vi "Configure Module.vi"(8 "error in (no error)":errorcluster, 10 "IOV ref in":variant, 11 "Modules.lvlib:9242.lvclass":refnum<class "9242.lvclass">) -> (0 "error out":errorcluster, 2 "IOV ref out":variant, 3 "Modules.lvlib:9242.lvclass":refnum<class "9242.lvclass">)   [LabVIEW 2020, in "Modules.lvlib" / "9242.lvclass"]
uses:
  9242.lvclass
  <resource>/objmgr/cRIO.rc
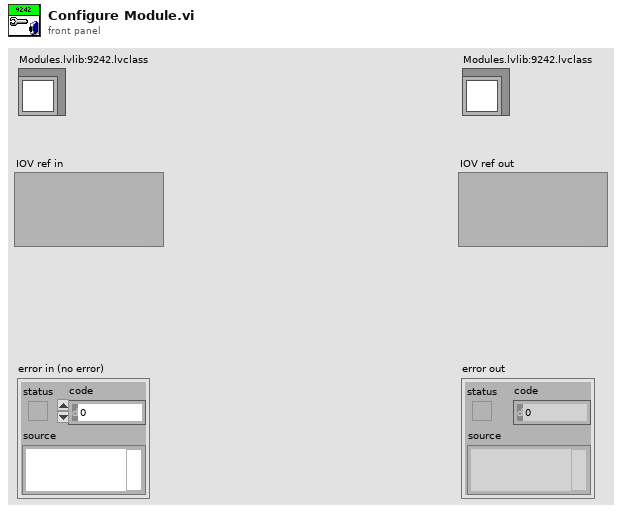
[diagram p1: front panel]
types:
  T1 = typedef "Modules.lvlib/9233.lvclass/Data rate.ctl" = u32
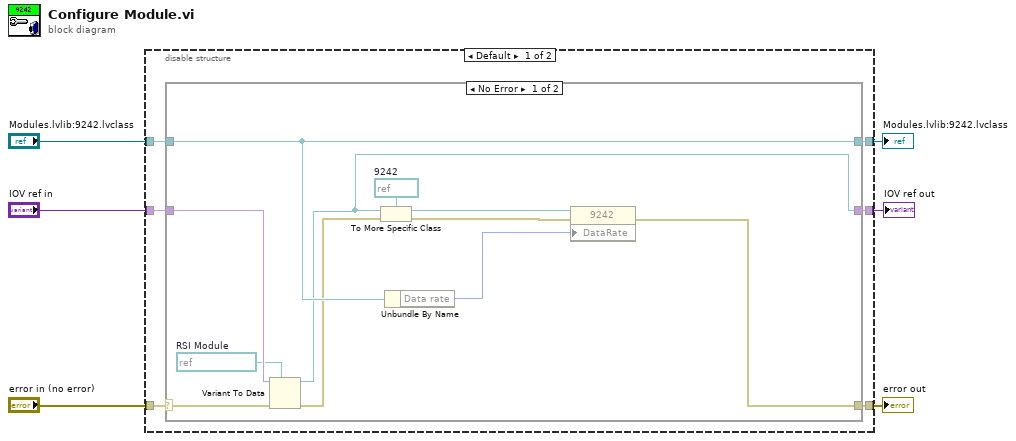
[diagram p0: block diagram]
diagram:
  n1 = disable-structure shown="Default" {
    disable-tunnel: "error in (no error)" -> [w12 w27]
    disable-tunnel: [w11 w27] -> w5
    disable-tunnel: "Modules.lvlib:9242.lvclass" -> [w10 w29]
    disable-tunnel: [w9 w29] -> w3
    disable-tunnel: "IOV ref in" -> [w8 w28]
    disable-tunnel: [w7 w28] -> w1
    frame condition #0 {
      n2 = case shown="No Error" w12 {
        selector: w12 -> [w22 w26]
        tunnel: [w18 w26] -> w11
        tunnel: [w23 w25] -> w9
        tunnel: w10 -> [w23 w25]
        tunnel: w8 -> [w15 w24]
        tunnel: [w14 w24] -> w7
        frame No Error {
          w13 = refnum<k21> refnum  # RSI Module
          w21 = refnum<k21> refnum  # 9242
          n3 = Variant To Data(error in=w22, type=w13, Variant=w15) -> (data=w14:refnum<k21>, error out=w16:errorcluster)
          n4 = To More Specific Class(target class=w21, reference=w14, error in=w16) -> (specific class reference=w20:refnum<k21>, error out=w19:errorcluster)
          n5 = Unbundle By Name(w23) -> ("Data rate"=w17:T1)
          n6 = property class="9242"(reference=w20, error in=w19, "DataRate"=w17) -> (error out=w18:errorcluster)  [unwired: 1 out]
        }
        frame Error {
        }
      }
    }
    frame condition #1 (active) {
    }
  }
  "error out" <- w5
  "Modules.lvlib:9242.lvclass" <- w3
  "IOV ref out" <- w1
